vi "RshTest.vi"() -> ()   [LabVIEW 2017]
uses:
  <vilib>/Utility/file.llb/Read Delimited Spreadsheet (DBL).vi
panel:
  out "Rsh":dbl
  in  "file path (dialog if empty)":path=path "C:/Users/Jonathan/Documents/UHasselt/Masterproef/LabVEIW/data/24-05-19_11h55/Module1/0.csv"
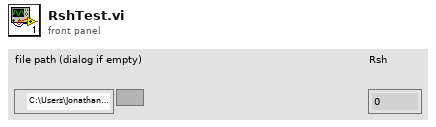
[diagram p1: front panel]
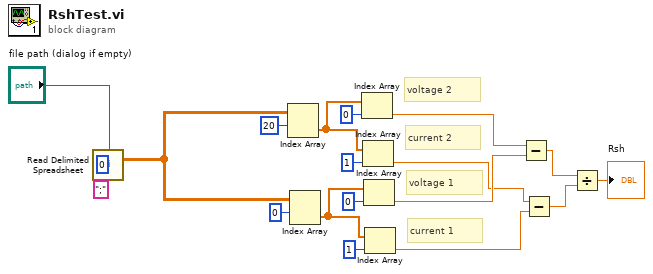
[diagram p0: block diagram]
diagram:
  # "current 1"
  # "voltage 1"
  # "current 2"
  # "voltage 2"
  n1 = call-poly <vilib>:"Read Delimited Spreadsheet.vi"("file path (dialog if empty)"="file path (dialog if empty)", "start of read offset (chars.:0)"=0, "delimiter (\\t)"=";" ("delimiter (\\t)")) -> ("all rows"=w15:dbl[][])  [unwired: 7 in, 5 out]
  n2 = Index Array(array=w15, index (row)=20) -> (element=w11:dbl[])  [unwired: 1 in]
  n3 = Index Array(array=w15, index (row)=0) -> (element=w8:dbl[])  [unwired: 1 in]
  n4 = Index Array(array=w11, index=0) -> (element=w4:dbl)
  n5 = Index Array(array=w11, index=1) -> (element=w2:dbl)
  n6 = Index Array(array=w8, index=0) -> (element=w3:dbl)
  n7 = Index Array(array=w8, index=1) -> (element=w1:dbl)
  n8 = Subtract(x=w4, y=w3) -> (x-y=w7:dbl)
  n9 = Subtract(x=w2, y=w1) -> (x-y=w6:dbl)
  n10 = Divide(x=w7, y=w6) -> (x/y=→"Rsh":dbl)
